vi "ConvertNumericString.vi"(2 "Input":string) -> (7 "Output":string)   [LabVIEW 2010]
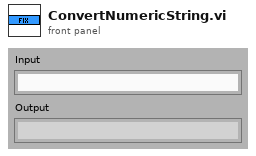
[diagram p1: front panel]
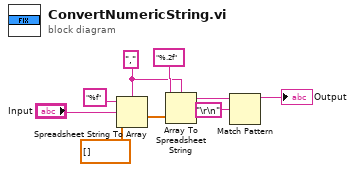
[diagram p0: block diagram]
diagram:
  w4 = "," ("delimiter (Tab)")
  n1 = Spreadsheet String To Array(delimiter (Tab)=w4, format string="%f", spreadsheet string="Input", array type (2D Dbl)=dbl[] []) -> (array=w6:dbl[])
  n2 = Array To Spreadsheet String(delimiter (Tab)=w4, array=w6, 3:"%.2f" ("format string")) -> (spreadsheet string=w3:string)
  n3 = Match Pattern(string=w3, regular expression="\r\n") -> (before substring=→"Output":string)  [unwired: 1 in, 3 out]
